vi "Gate sweep_S.vi"() -> ()   [LabVIEW 2012]
uses:
  <vilib>/express/express arith-compare/Formula/XNode/ExpressFormulaBlockNode.xnode
panel:
  in  "Measure Infos":string="Sample: XXX"
  in  "Voltage":cluster{"V-start":dbl, "Step":ext, "V-end":dbl}={"V-start"=0.0, "Step"=0.1, "V-end"=2.0} {"Step" format="%#.6f"; "V-start" format="%#.2f"}
  in  "Instr Adress":T1={"Keithley"="18", "Lockin 1"="8", "Lockin 2"="9", "Lockin 3"="10", "Keithley Label"="Current", "Lockin 1 Label "="Vxx", "Lockin2 Label"="Vxy", "Lockin3 Label"="Vxy"}
  out "Current":cluster{"Y":dbl[], "Y":dbl[]}[](graph)
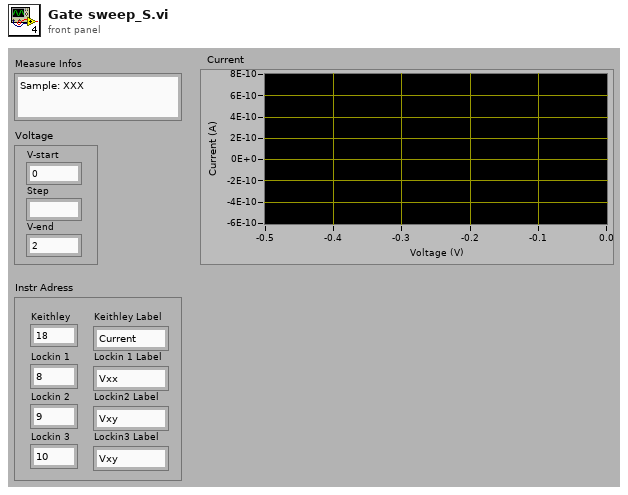
[diagram p1: front panel]
types:
  T1 = cluster{"Keithley":string, "Lockin 1":string, "Lockin 2":string, "Lockin 3":string, "Keithley Label":string, "Lockin 1 Label ":string, "Lockin2 Label":string, "Lockin3 Label":string}
  T2 = enum16{"open", "replace", "create", "open or create", "replace or create", "replace or create with confirmation"}
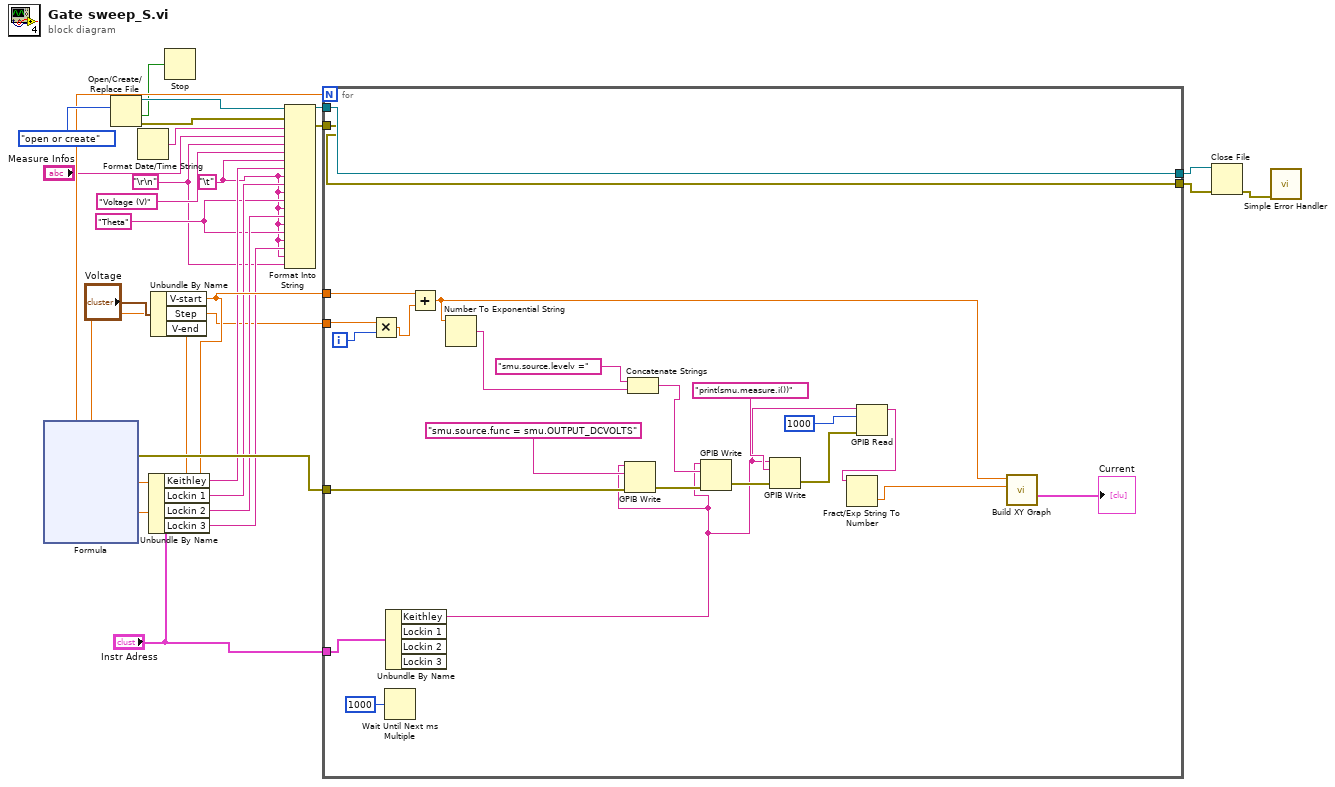
[diagram p0: block diagram]
diagram:
  w6 = "Theta"
  w4 = "\t"
  w3 = "\r\n"
  n1 = Open/Create/Replace File(operation (0:open)=T2."open or create") -> (refnum out=w17:refnum<file>, cancelled=w2:bool, error out=w15:errorcluster)  [unwired: 5 in]
  n2 = Format Date/Time String() -> (date/time string=w13:string)  [unwired: 3 in]
  n3 = Unbundle By Name("Instr Adress") -> ("Keithley"=w9:string, "Lockin 1"=w8:string, "Lockin 2"=w7:string, "Lockin 3"=w5:string)
  n4 = Unbundle By Name("Voltage") -> ("V-start"=w24:dbl, "Step"=w1:ext, "V-end"=w23:dbl)
  n5 = xnode ("Formula")("Vend"=w23, "Vstart"=w24, "step"=w1) -> ("Result"=w19:ext, "error out"=w26:errorcluster)  [unwired: 1 in]
  n6 = Stop(stop? (T)=w2) -> ()
  n7 = Format Into String(initial string=w17, error in=w15, w13, "Measure Infos", w3, "Voltage (V)", w4, w9, w4, w8, w4, w6, w4, w7, w4, w6, w4, w5, w4, w3) -> (resulting string=w16:refnum<file>, error out=w14:errorcluster)  [unwired: 1 in]
  n8 = for {
    N: w19 -> [_]
    tunnel: w26 -> [w37]
    tunnel: w1 -> [w34]
    tunnel: w24 -> [w44]
    tunnel: "Instr Adress" -> [w32]
    tunnel: w16 -> [w28]
    tunnel: w14 -> [w27]
    tunnel: [w28] -> w22
    tunnel: [w27] -> w21
    i -> [w46]
    n9 = Multiply(x=w34, y=w46) -> (x*y=w43:ext)
    n10 = Wait Until Next ms Multiple(millisecond multiple=u32 1000) -> ()  [unwired: 1 out]
    n11 = Unbundle By Name(w32) -> ("Keithley"=w31:string)  [unwired: 3 out]
    n12 = Add(x=w44, y=w43) -> (x+y=w30:ext)
    n13 = Number To Exponential String(number=w30) -> (E-format string=w47:string)  [unwired: 3 in]
    n14 = GPIB Write(0:w31, 1:"smu.source.func = smu.OUTPUT_DCVOLTS" ("write buffer"), 3:w37) -> (6:w38:errorcluster)  [unwired: 2 in, 1 out]
    n15 = Concatenate Strings("smu.source.levelv =", w47) -> (w41:string)
    n16 = GPIB Write(0:w31, 1:w41, 3:w38) -> (6:w39:errorcluster)  [unwired: 2 in, 1 out]
    n17 = GPIB Write(0:w31, 1:"print(smu.measure.i())", 3:w39) -> (6:w33:errorcluster)  [unwired: 2 in, 1 out]
    n18 = GPIB Read(0:w31, 1:u32 1000 ("byte count"), 3:w33) -> (5:w36:string)  [unwired: 2 in, 2 out]
    n19 = Fract/Exp String To Number(string=w36) -> (number=w29:dbl)  [unwired: 3 in, 1 out]
    n20 = call "Build XY Graph"("Y Input"=w29, "X Input"=w30) -> ("XY Graph"=→"Current":cluster{"Y":dbl[], "Y":dbl[]}[])  [unwired: 8 in, 1 out]
  }
  n21 = Close File(refnum=w22, error in=w21) -> (error out=w18:errorcluster)  [unwired: 1 out]
  n22 = call <vilib>:"Simple Error Handler.vi"("error in (no error)"=w18) -> ()  [unwired: 4 in, 5 out]
